vi "Memory Management.MoveByteBlock.Read (Double).vi"(0 "src in":dbl[](array[numeric]), 1 "src offset (0)":u64, 2 "dst ptr in":u64, 3 "dst offset (0)":u64, 4 "size":i64, 5 "error in (no error)":errorcluster) -> (14 "src out":dbl[](array[numeric]), 15 "src offset out":u64, 16 "dst ptr out":u64, 17 "dst offset out":u64, 18 "size out":i64, 19 "error out":errorcluster)   [LabVIEW 2016, in "VeriStand Data.lvlib"]
doc: "Calls into VeriStand's Data Services library to move a data block of length <B>size</B> from the <B>src</B> to <B>dst</B>."
uses:
  VeriStand Data.lvlib
  <vilib>/NI Veristand/Custom Device API/data/NIVeriStand_DataServices.dll
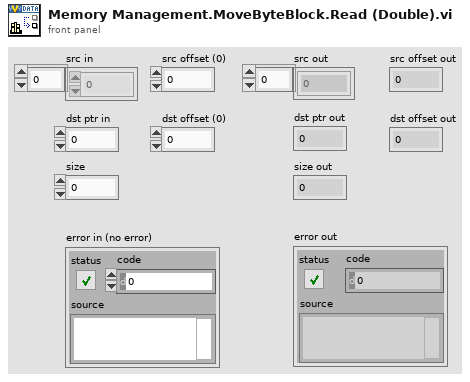
[diagram p1: front panel]
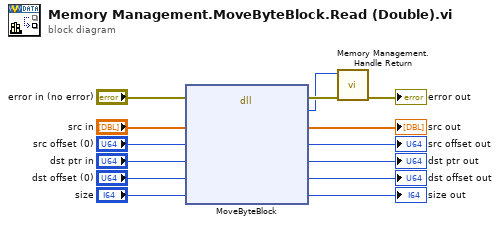
[diagram p0: block diagram]
diagram:
  n1 = dll-call lib="C:/Program Files (x86)/National Instruments/LabVIEW 2016/vi.lib/NI Veristand/Custom Device API/data/NIVeriStand_DataServices.*" fn="MoveByteBlock"(error in="error in (no error)", "srcPtr"="src in", "srcOffset"="src offset (0)", "dstPtr"="dst ptr in", "dstOffset"="dst offset (0)", "size"="size") -> (error out=w10:errorcluster, "return type"=w8:i32, "srcPtr"=→"src out":dbl[], "srcOffset"=→"src offset out":u64, "dstPtr"=→"dst ptr out":u64, "dstOffset"=→"dst offset out":u64, "size"=→"size out":i64)  [unwired: 2 in, 1 out]
  n2 = call "Memory Management.Handle Return.vi"("error in (no error)"=w10, "return"=w8) -> ("error out"=→"error out":errorcluster)  [unwired: 9 in]
